vi "On Success.vi"(8 "error in (no error)":errorcluster, 9 "Session In":refnum<class "Session.lvclass">, 10 "User":refnum<class "User.lvclass">, 11 "Authentication Provider in":refnum<class "Authentication Provider.lvclass">) -> (0 "error out":errorcluster, 1 "Session":refnum<class "Session.lvclass">, 2 "Response":refnum<class "Response.lvclass">, 3 "Authentication Provider out":refnum<class "Authentication Provider.lvclass">)   [LabVIEW 2020, in "HTTP Server.lvlib" / "Authentication Provider.lvclass"]
uses:
  Authentication Provider.lvclass
  lv-http-util/HTTP Utils/Response/Response.lvclass
  Session/Session.lvclass
  User/User.lvclass
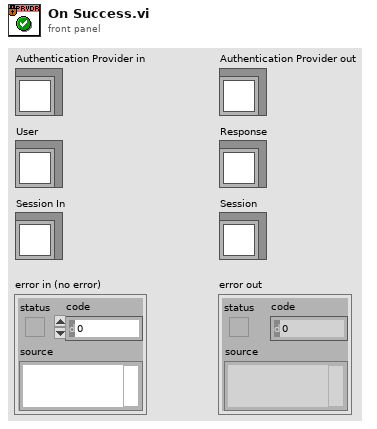
[diagram p1: front panel]
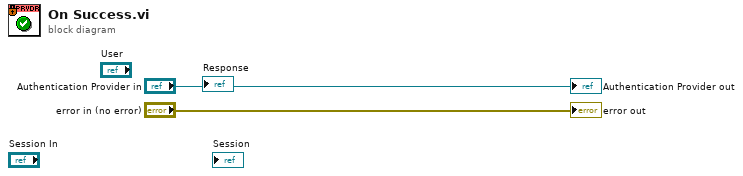
[diagram p0: block diagram]
diagram:
  "error out" <- "error in (no error)"
  "Authentication Provider out" <- "Authentication Provider in"
